vi "Constructor.vi"(0 "DBSet in":refnum<class "DBSet.lvclass">, 1 "SQLite DB Path":path, 11 "error in (no error)":errorcluster {"code" format="Error %.0f"}) -> (4 "DBSet out":refnum<class "DBSet.lvclass">, 15 "error out":errorcluster {"code" format="Error %.0f"})   [LabVIEW 2024, in "DBSet.lvclass"]
uses:
  DBSet.lvclass
  DBSet.lvclass/DBSet.ctl
  <vilib>/drjdpowell/SQLite Library/SQL Connection/Open (string).vi
  <vilib>/drjdpowell/SQLite Library/SQL Connection/Execute SQL (No results).vi
  <vilib>/drjdpowell/SQLite Library/SQL Connection/Connection.lvclass
  <vilib>/drjdpowell/SQLite Library/SQLite.lvlib
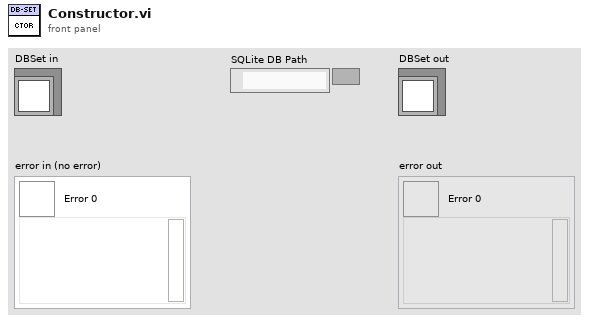
[diagram p1: front panel]
types:
  T1 = enum16{"New or existing", "Existing", "Read only"}
  T2 = typedef "Semaphore RefNum" = refnum<k1>
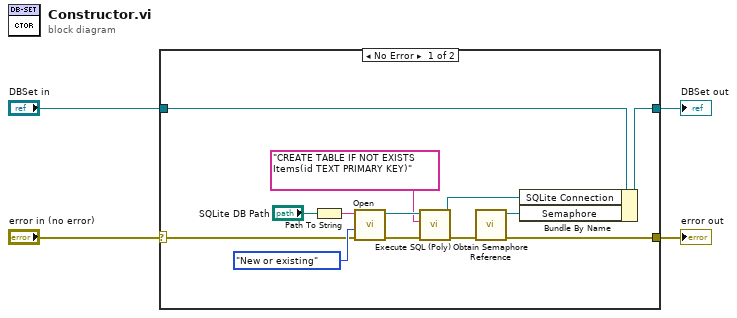
[diagram p0: block diagram]
diagram:
  n1 = case shown="No Error" "error in (no error)" {
    selector: "error in (no error)" -> [w11 w19]
    tunnel: [w8 w19] -> w3
    tunnel: [w6 w18] -> w1
    tunnel: "DBSet in" -> [w5 w18]
    frame No Error {
      n2 = Path To String(path="SQLite DB Path") -> (string=w17:string)
      n3 = call-poly <vilib>:"Open.vi"("error in (no error)"=w11, "File Option"=T1."New or existing", "db file"=w17) -> ("error out"=w16:errorcluster, "SQLite Connection"=w15:refnum<class "Connection.lvclass">)  [unwired: 7 in]
      n4 = call-poly <vilib>:"Execute SQL (Poly).vi"("error in (no error)"=w16, "SQL"="CREATE TABLE IF NOT EXISTS Items(id TEXT PRIMARY KEY)", "SQLite Connection in"=w15) -> ("error out"=w9:errorcluster, "SQLite Connection"=w7:refnum<class "Connection.lvclass">)  [unwired: 7 in]
      n5 = call <vilib>:"Obtain Semaphore Reference.vi"("error in (no error)"=w9) -> ("error out"=w8:errorcluster, "semaphore"=w10:T2)  [unwired: 4 in, 1 out]
      n6 = Bundle By Name(cluster=w5, "SQLite Connection"=w7, "Semaphore"=w10) -> (w6:refnum<class "DBSet.lvclass">)
    }
    frame Error {
    }
  }
  "error out" <- w3
  "DBSet out" <- w1
